vi "Mobus Master3.vi"() -> ()   [LabVIEW 2015]
uses:
  <vilib>/Modbus/master/Create Master Instance (Serial).vi
  <vilib>/Modbus/master/Modbus Master.lvclass
panel:
  out "LED 2":bool
  out "LDR 2":dbl(slide) scale=0.0..5.0
  out "LDR 1":dbl(slide) scale=0.0..5.0
  in  "stop":bool
  out "LED 1":bool
  out "LED 2":u16
  out "LED 1":u16
  out "LDR 2":dbl
  out "LDR 1":dbl
  out "Read Register":u16[](array[numeric])
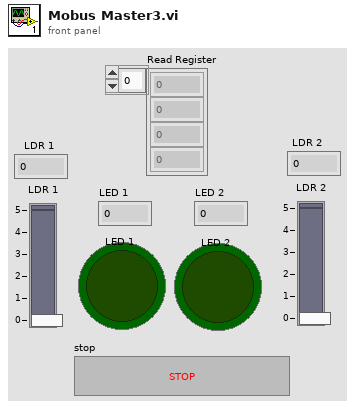
[diagram p1: front panel]
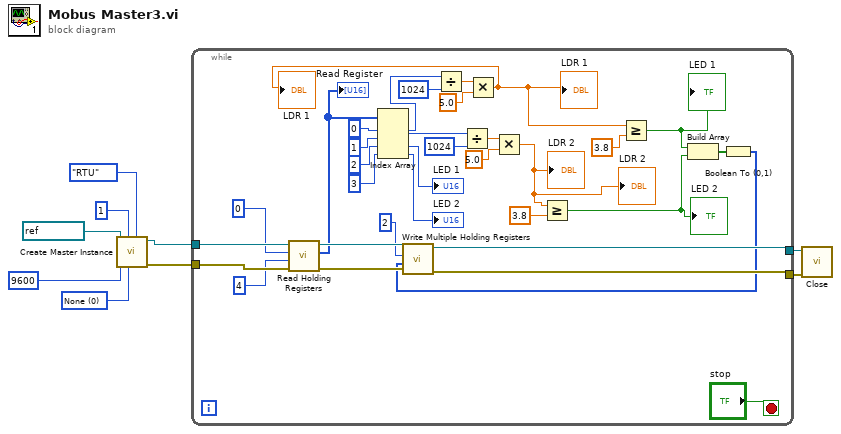
[diagram p0: block diagram]
diagram:
  w1 = u16 0 items=["None", "Odd", "Even"] ("parity (Even)")
  n1 = call-poly <vilib>:"Create Master Instance.vi"("serial type"=enum16{"RTU", "ASCII"}."RTU", "parity (Even)"=w1, "unit ID"=u8 1, "baud rate (9600)"=u32 9600, "VISA resource name"=refnum<visa-resource-name> "COM9") -> ("error out"=w7:errorcluster, "serial master instance"=w9:refnum<class "Modbus Master.lvclass">)  [unwired: 5 in]
  n2 = while {
    tunnel: w9 -> [w42]
    tunnel: [w37] -> w8
    tunnel: w7 -> [w41]
    tunnel: [w35] -> w6
    stop <- "stop" stop-if-true
    n3 = call-dynamic "Read Holding Registers.vi"("error in (no error)"=w41, "number of holding registers"=u16 4, "starting address"=u16 0, "Modbus master in"=w42) -> ("error out"=w36:errorcluster, "register values"=w33:u16[], "Modbus master out"=w38:refnum<class "Modbus Master.lvclass">)  [unwired: 5 in]
    "Read Register" <- w33
    n4 = Index Array(array=w33, index #1=0 ("index"), index #2=1 ("index"), index #3=2 ("index"), index #4=3 ("index")) -> (element #1=w28:u16, element #2=w21:u16, element #3=→"LED 1":u16, element #4=→"LED 2":u16)
    n5 = Divide(x=w28, y=u16 1024 ("x")) -> (x/y=w26:dbl)
    n6 = Divide(x=w21, y=u16 1024 ("x")) -> (x/y=w23:dbl)
    n7 = Multiply(x=w26, y=5.0) -> (x*y=w12:dbl)
    "LDR 1" <- w12
    "LDR 1" <- w12
    n8 = Multiply(x=w23, y=5.0) -> (x*y=w11:dbl)
    "LDR 2" <- w11
    "LDR 2" <- w11
    n9 = Greater Or Equal?(x=w11, y=3.8) -> (x >= y?=w10:bool)
    "LED 2" <- w10
    n10 = Greater Or Equal?(x=w12, y=3.8) -> (x >= y?=w16:bool)
    "LED 1" <- w16
    n11 = Build Array(w16, w10) -> (w15:bool[])
    n12 = Boolean To (0,1)(Boolean=w15) -> (0, 1=w14:i16[])
    n13 = call-dynamic "Write Multiple Holding Registers.vi"("error in (no error)"=w36, "holding register values"=w14, "starting address"=u16 2, "Modbus master in"=w38) -> ("error out"=w35:errorcluster, "Modbus master out"=w37:refnum<class "Modbus Master.lvclass">)  [unwired: 6 in]
  }
  n14 = call-dynamic "Close.vi"("error in (no error)"=w6, "Modbus master in"=w8) -> ()  [unwired: 9 in, 1 out]
